vi "Register Message Metadata.vi"(8 "error in":errorcluster, 10 "Messages":T2[](array[typedef]), 11 "gRPCid in":T1) -> (0 "error out":errorcluster, 3 "gRPCid out":T1)   [LabVIEW 2019, in "grpc-lvsupport.lvlib"]
uses:
  grpc-lvsupport.lvlib
  Message Metadata.ctl
  Message Element Metadata.ctl
  Message Element Type.ctl
  grpcId.ctl
  <vilib>/Utility/file.llb/Application Directory.vi
  <vilib>/Utility/error.llb/Error Cluster From Error Code.vi
  <resource>/labview_grpc_server.dll
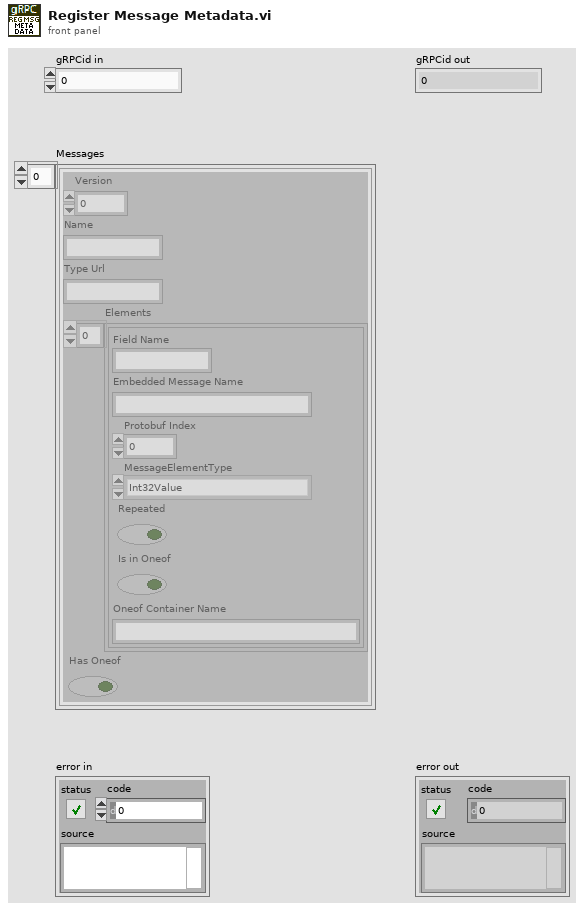
[diagram p1: front panel]
types:
  T1 = typedef "grpc-lvsupport.lvlib/grpcId.ctl" = u64
  T2 = typedef "grpc-lvsupport.lvlib/Message Metadata.ctl" = cluster{"Version":i32, "Name":string, "Type Url":string, "Elements":T3[], "Has Oneof":bool}
  T3 = typedef "grpc-lvsupport.lvlib/Message Element Metadata.ctl" = cluster{"Field Name":string, "Embedded Message Name":string, "Protobuf Index":i32, "MessageElementType":T4, "Repeated":bool, "Is in Oneof":bool, "Oneof Container Name":string}
  T4 = typedef "grpc-lvsupport.lvlib/Message Element Type.ctl" = enum32{"Int32Value", "FloatValue", "DoubleValue", "BoolValue", "StringValue", "MessageValue", "Int64Value", "UInt32Value", "UInt64Value", "EnumValue", "Bytes", "Fixed64", "Fixed32", "SFixed64", "SFixed32", "SInt64", "SInt32"}
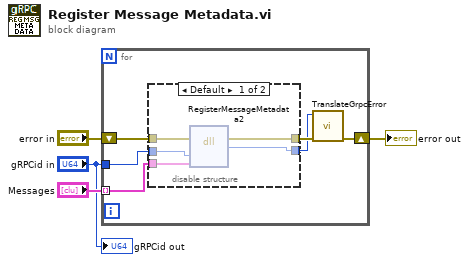
[diagram p0: block diagram]
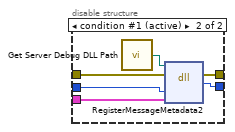
[diagram p2: hidden frame]
diagram:
  n1 = for {
    tunnel: "Messages" -> [w8] mode=indexing
    shift-right: [w7] -> w2
    shift-left: "error in" -> [w10]
    tunnel: "gRPCid in" -> [w5]
    n2 = disable-structure shown="Default" {
      disable-tunnel: w10 -> [w15 w21]
      disable-tunnel: [w14 w20] -> w9
      disable-tunnel: w8 -> [w13 w19]
      disable-tunnel: w5 -> [w11 w18]
      disable-tunnel: [w12 w17] -> w6
      frame condition #0 {
        n3 = dll-call lib="C:/Program Files (x86)/National Instruments/LabVIEW 2024/resource/labview_grpc_server.*" fn="RegisterMessageMetadata2"(error in=w15, "serverId"=w11, "metadata"=w13) -> (error out=w14:errorcluster, "return type"=w12:i32)  [unwired: 4 in, 1 out]
      }
      frame condition #1 (active) {
        n4 = call "Get Server Debug DLL Path.vi"() -> ("DLL Path"=w16:path)
        n5 = dll-call lib="?" fn="RegisterMessageMetadata2"(path in=w16, error in=w21, "serverId"=w18, "metadata"=w19) -> (error out=w20:errorcluster, "return type"=w17:i32)  [unwired: 3 in, 1 out]
      }
    }
    n6 = call "TranslateGrpcError.vi"("error in"=w9, "Error Code"=w6) -> ("error out"=w7:errorcluster)  [unwired: 9 in]
  }
  "error out" <- w2
  "gRPCid out" <- "gRPCid in"
